vi "Disable Unavailable Channels.vi"(8 "error in (no error)":errorcluster, 10 "Item Ref out":T1 format="%.0x", 11 "Ring in":refnum<vi>) -> (0 "error out":errorcluster)   [LabVIEW 2011, in "Simulated Thermocouple Custom Device.lvlib"]
uses:
  Simulated Thermocouple Custom Device.lvlib
  <vilib>/NI Veristand/Custom Device API/Custom Device Item Ref.ctl
  <vilib>/NI Veristand/Custom Device API/Custom Device API.lvlib
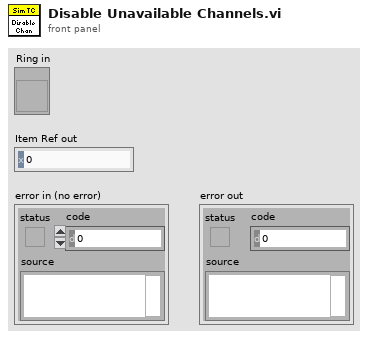
[diagram p1: front panel]
types:
  T1 = typedef "Custom Device API.lvlib/Custom Device Item Ref.ctl" = u64
  T2 = typedef "Simulated Thermocouple Custom Device.lvlib/Device Config data.ctl" = cluster{"Custom Device Ref":T1, "Voltage Section Ref":T1, "simTC Section Refs":T1[], "Current Section Ref":T1, "Physical Device":string, "Available Physical Channels":i32[], "Channel Counts":u32[], "Dev Chan Count":u32}
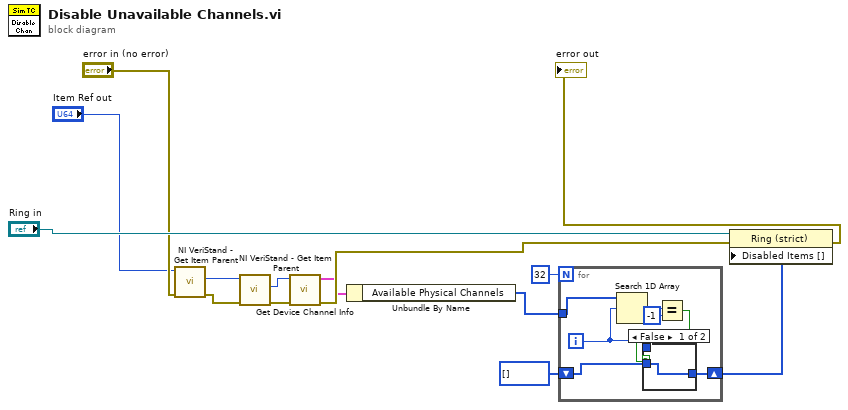
[diagram p0: block diagram]
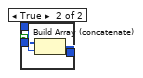
[diagram p2: hidden frame]
diagram:
  n1 = call <vilib>:"NI VeriStand - Get Item Parent.vi"("error in (no error)"="error in (no error)", "Item Ref in"="Item Ref out") -> ("error out"=w5:errorcluster, "Parent Ref"=w2:T1)  [unwired: 6 in, 2 out]
  n2 = call <vilib>:"NI VeriStand - Get Item Parent.vi"("error in (no error)"=w5, "Item Ref in"=w2) -> ("error out"=w6:errorcluster, "Parent Ref"=w1:T1)  [unwired: 6 in, 2 out]
  n3 = call "Get Device Channel Info.vi"("error in"=w6, "Custom Device Ref in"=w1) -> ("error out"=w8:errorcluster, "Device Configuration Data"=w7:T2)  [unwired: 7 in, 1 out]
  n4 = Unbundle By Name(w7) -> ("Available Physical Channels"=w11:i32[])
  n5 = for {
    N: 32 -> [_]
    tunnel: w11 -> [w21]
    shift-right: [w18] -> w13
    shift-left: i32[] [] ("Available Physical Channels") -> [w19]
    i -> [w20]
    n6 = Search 1D Array(1D array=w21, element=w20) -> (index of element=w17:i32)  [unwired: 1 in]
    n7 = Equal?(x=w17, y=-1) -> (x = y?=w15:bool)
    n8 = case shown="False" w15 {
      tunnel: w20 -> [_ w25]
      tunnel: w19 -> [w22 w24]
      tunnel: [w22 w23] -> w18
      frame False {
      }
      frame True {
        n9 = Build Array (concatenate)(w24, w25) -> (w23:i32[])
      }
    }
  }
  n10 = property class="Ring (strict)"(reference="Ring in", error in=w8, "Disabled Items []"=w13) -> (error out=→"error out":errorcluster)  [unwired: 1 out]
